vi "Write Data.vi"(8 "error in (no error)":errorcluster, 9 "Publication Time":timestamp, 10 "Value":variant, 11 "ConfigurationFileBinding In":refnum<class "ConfigurationFileBinding.lvclass">) -> (0 "error out":errorcluster, 3 "ConfigurationFileBinding Out":refnum<class "ConfigurationFileBinding.lvclass">)   [LabVIEW 2020, in "ConfigurationFileBinding.lvclass"]
doc: "<License>\nCopyright © 2017 Composed Systems, LLC | All rights reserved\nwww.composed.io\n\nAuthor: Ethan Stern <ethan.stern@composed.io>\n\nThis software is provided \"AS IS\" WITHOUT WARRANTIES, either express or implied, AND IS FOR EDUCATIONAL PURPOSES ONLY.\n</License>"
uses:
  <vilib>/gpm_packages/@cs/transport/Source/Concrete/ConfigurationFileBinding/ConfigurationFileBinding.lvclass
  <vilib>/gpm_packages/@cs/transport/Source/Concrete/ConfigurationFileBinding/ConfigurationFileBinding.lvclass/ConfigurationFileBinding.ctl
  <vilib>/Utility/error.llb/Error Cluster From Error Code.vi
  <vilib>/Utility/config.llb/Write Key (I32).vi
  <vilib>/Utility/config.llb/Write Key (U32).vi
  <vilib>/Utility/config.llb/Write Key (Double).vi
  <vilib>/Utility/config.llb/Write Key (Boolean).vi
  <vilib>/Utility/config.llb/Write Key (String).vi
  <vilib>/Utility/config.llb/Write Key (Path).vi
  <vilib>/ErrorRing/Error Ring.xnode
  <vilib>/Utility/Data Type/NI_Data Type.lvlib
  <vilib>/Utility/config.llb/NI_LVConfig.lvlib
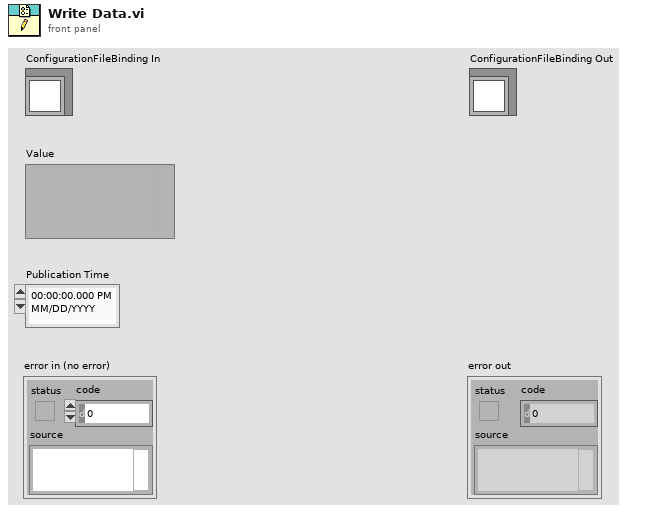
[diagram p1: front panel]
types:
  T1 = typedef "NI_LVConfig.lvlib/Config Data RefNum.ctl" = refnum<k1>
  T2 = typedef "NI_Data Type.lvlib/Data Type.ctl" = enum8{"Invalid Type", "Void", "I8", "I16", "I32", "I64", "U8", "U16", "U32", "U64", "Single Float", "Double Float", "Extended Float", "Single Complex", "Double Complex", "Extended Complex", "Enum U8", "Enum U16", "Enum U32", "Enum U64", "Single Float With Unit", "Double Float With Unit", "Extended Float With Unit", "Single Complex with Unit", "Double Complex with Unit", "Extended Complex with Unit", "Boolean", "String", "Path", "Picture", "Tag", "Array", "Cluster", "Variant", "LV Variant", "Waveform", "Timestamp", "Digital Waveform", "Digital Data", "ExpressData", "Refnum", "External Data", "VI", "Poly VI", "LabVIEW Class Instance", "Fixed Point", "Set Collection", "Map Collection"}
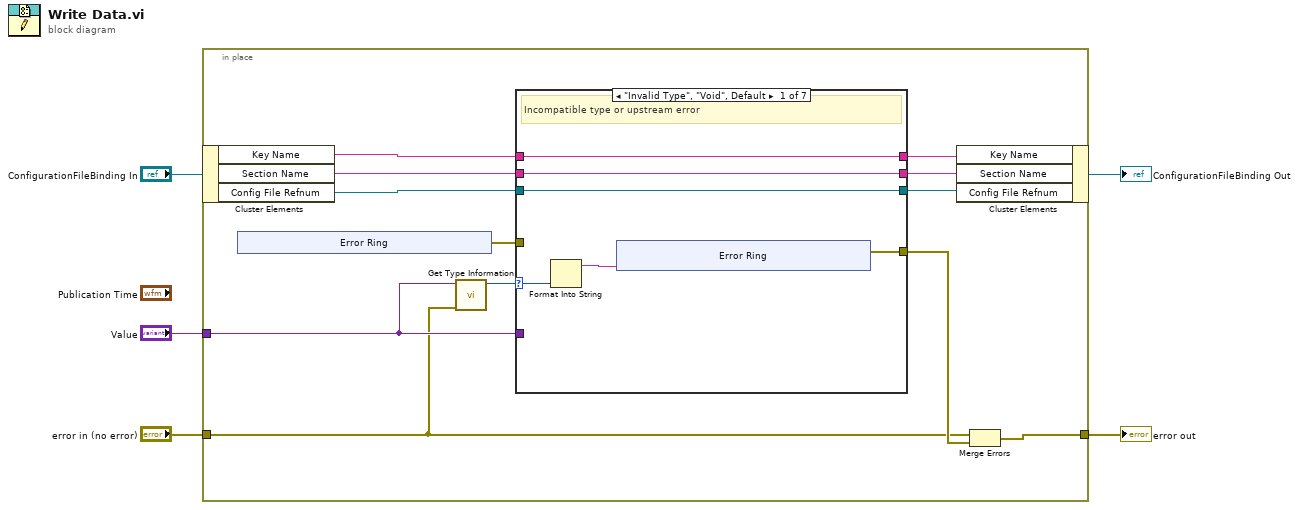
[diagram p0: block diagram]
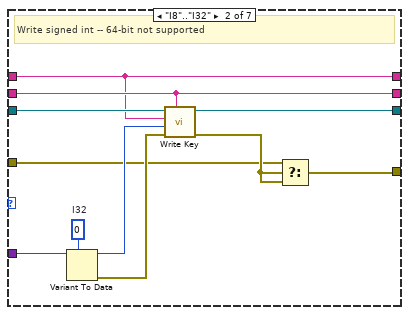
[diagram p2: hidden frame]
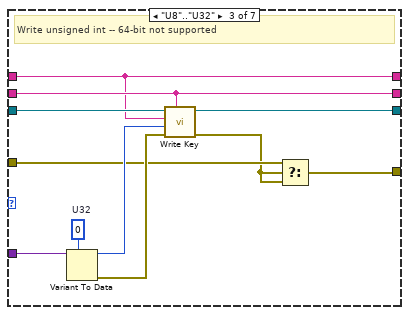
[diagram p3: hidden frame]
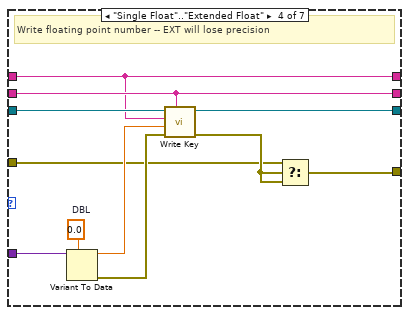
[diagram p4: hidden frame]
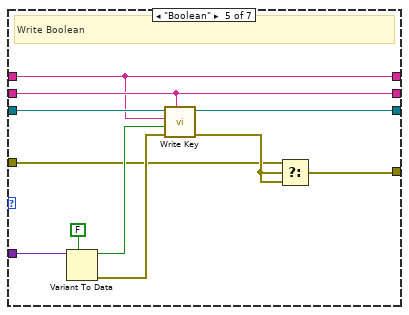
[diagram p5: hidden frame]
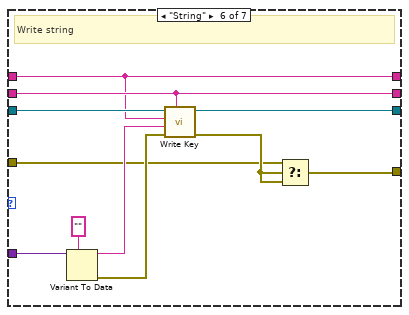
[diagram p6: hidden frame]
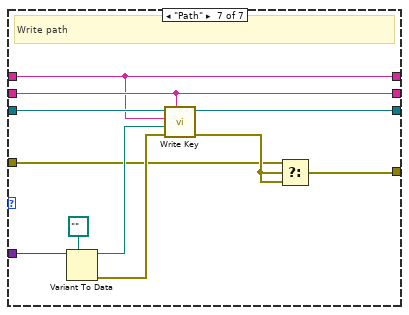
[diagram p7: hidden frame]
diagram:
  n1 = in-place {
    in-place-border: [w17] -> w5
    in-place-border: "Value" -> [w15]
    in-place-border: "error in (no error)" -> [w13]
    n2 = in-place-cluster #1("ConfigurationFileBinding In") -> ("Key Name"=w8:string, "Section Name"=w10:string, "Config File Refnum"=w11:T1)
    n3 = xnode "Error Ring"() -> ("error out"=w6:errorcluster)
    n4 = call <vilib>:"Get Type Information.vi"("error in (no error)"=w13, "variant"=w15) -> ("type"=w14:T2)  [unwired: 5 in, 4 out]
    n5 = case shown="\"Invalid Type\", \"Void\", Default" w14 {
      selector: w14 -> [w24 _ _ _ _ _ _]
      tunnel: [w28 w38 w49 w60 w70 w81 w92] -> w16
      tunnel: w15 -> [_ w45 w56 w67 w78 w89 w100]
      tunnel: [w27 w42 w53 w64 w75 w86 w97] -> w12
      tunnel: w11 -> [w27 w41 w52 w63 w74 w85 w96]
      tunnel: w10 -> [w26 w40 w51 w62 w73 w84 w95]
      tunnel: [w26 w40 w51 w62 w73 w84 w95] -> w9
      tunnel: w8 -> [w25 w39 w50 w61 w72 w83 w94]
      tunnel: [w25 w39 w50 w61 w72 w83 w94] -> w7
      tunnel: w6 -> [_ w36 w48 w58 w69 w80 w91]
      frame "Invalid Type", "Void", Default {
        # "Incompatible type or upstream error"
        n6 = Format Into String(w24) -> (resulting string=w23:string)  [unwired: 3 in, 1 out]
        n7 = xnode "Error Ring"("parameter 0"=w23) -> ("error out"=w28:errorcluster)
      }
      frame "I8".."I32" {
        w46 = 0  # I32
        # "Write signed int -- 64-bit not supported"
        n8 = Variant To Data(type=w46, Variant=w45) -> (data=w43:i32, error out=w44:errorcluster)  [unwired: 1 in]
        n9 = call-poly <vilib>:"Write Key.vi"("section"=w40, "error in (no error)"=w44, "value"=w43, "key"=w39, "refnum"=w41) -> ("error out"=w37:errorcluster, "refnum out"=w42:T1)  [unwired: 4 in, 1 out]
        n10 = Select(t=w36, s=w37, f=w37) -> (s? t:f=w38:errorcluster)
      }
      frame "U8".."U32" {
        w57 = u32 0  # U32
        # "Write unsigned int -- 64-bit not supported"
        n11 = Variant To Data(type=w57, Variant=w56) -> (data=w54:u32, error out=w55:errorcluster)  [unwired: 1 in]
        n12 = call-poly <vilib>:"Write Key.vi"("section"=w51, "error in (no error)"=w55, "value"=w54, "key"=w50, "refnum"=w52) -> ("error out"=w47:errorcluster, "refnum out"=w53:T1)  [unwired: 4 in, 1 out]
        n13 = Select(t=w48, s=w47, f=w47) -> (s? t:f=w49:errorcluster)
      }
      frame "Single Float".."Extended Float" {
        w68 = 0.0  # DBL
        # "Write floating point number -- EXT will lose precision"
        n14 = Variant To Data(type=w68, Variant=w67) -> (data=w65:dbl, error out=w66:errorcluster)  [unwired: 1 in]
        n15 = call-poly <vilib>:"Write Key.vi"("section"=w62, "error in (no error)"=w66, "value"=w65, "key"=w61, "refnum"=w63) -> ("error out"=w59:errorcluster, "refnum out"=w64:T1)  [unwired: 4 in, 1 out]
        n16 = Select(t=w58, s=w59, f=w59) -> (s? t:f=w60:errorcluster)
      }
      frame "Boolean" {
        # "Write Boolean"
        n17 = Variant To Data(type=FALSE, Variant=w78) -> (data=w76:bool, error out=w77:errorcluster)  [unwired: 1 in]
        n18 = call-poly <vilib>:"Write Key.vi"("section"=w73, "error in (no error)"=w77, "value"=w76, "key"=w72, "refnum"=w74) -> ("error out"=w71:errorcluster, "refnum out"=w75:T1)  [unwired: 4 in, 1 out]
        n19 = Select(t=w69, s=w71, f=w71) -> (s? t:f=w70:errorcluster)
      }
      frame "String" {
        # "Write string"
        n20 = Variant To Data(type="", Variant=w89) -> (data=w87:string, error out=w88:errorcluster)  [unwired: 1 in]
        n21 = call-poly <vilib>:"Write Key.vi"("section"=w84, "error in (no error)"=w88, "value"=w87, "key"=w83, "refnum"=w85) -> ("error out"=w82:errorcluster, "refnum out"=w86:T1)  [unwired: 4 in, 1 out]
        n22 = Select(t=w80, s=w82, f=w82) -> (s? t:f=w81:errorcluster)
      }
      frame "Path" {
        # "Write path"
        n23 = Variant To Data(type=path "", Variant=w100) -> (data=w98:path, error out=w99:errorcluster)  [unwired: 1 in]
        n24 = call-poly <vilib>:"Write Key.vi"("section"=w95, "error in (no error)"=w99, "value"=w98, "key"=w94, "refnum"=w96) -> ("error out"=w93:errorcluster, "refnum out"=w97:T1)  [unwired: 4 in, 1 out]
        n25 = Select(t=w91, s=w93, f=w93) -> (s? t:f=w92:errorcluster)
      }
    }
    n26 = in-place-cluster #1("Key Name"=w7, "Section Name"=w9, "Config File Refnum"=w12) -> (→"ConfigurationFileBinding Out":refnum<class "ConfigurationFileBinding.lvclass">)
    n27 = Merge Errors(w13, w16) -> (w17:errorcluster)
  }
  "error out" <- w5
